vi "CompileReadHDF5PulseSeq.vi"(11 "path":path) -> (2 "parameter_config":string, 3 "pulse_seq_out":string)   [LabVIEW 2019]
uses:
  <vilib>/UPVI/lvhdf5/file.llb/LVH5F Operation.ctl
  <vilib>/UPVI/lvhdf5/group.llb/OpenCreateGroup (String).vi
  <vilib>/UPVI/lvhdf5/attribute.llb/Simple H5Aread (Variant).vi
  <vilib>/UPVI/lvhdf5/Attribute.llb/Simple H5Aread.xnode
  <vilib>/UPVI/lvhdf5/library.llb/HDF5 Ref.ctl
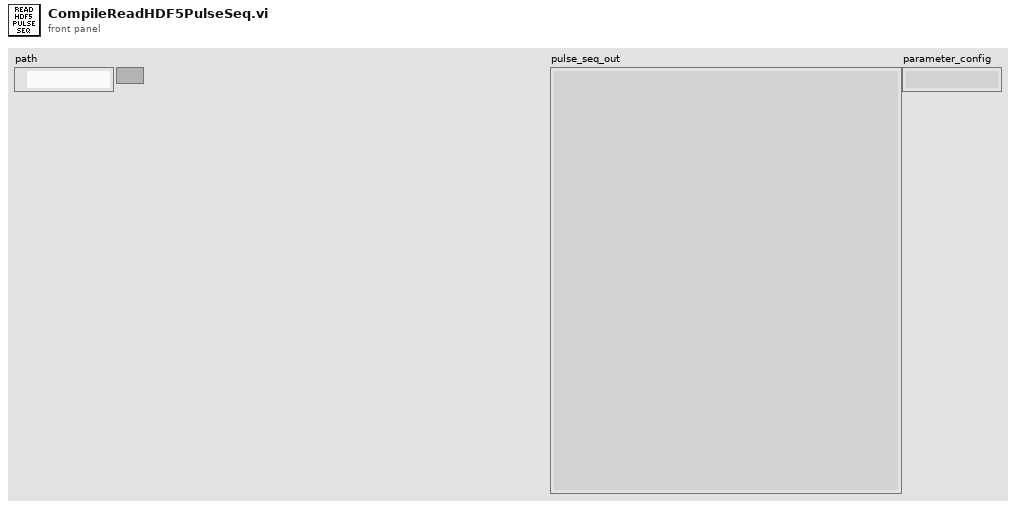
[diagram p1: front panel]
types:
  T1 = typedef "LVH5F Operation.ctl" = enum16{"open", "open or create", "create or replace", "create or replace (with confirmation)", "create", "open (read only)"}
  T2 = typedef "HDF5 Ref.ctl" = refnum<k1>
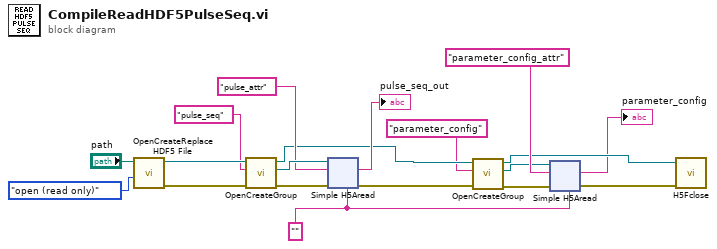
[diagram p0: block diagram]
diagram:
  w2 = ""
  n1 = call <vilib>:"OpenCreateReplace HDF5 File.vi"("function (open or create)"=LVH5F_Operation."open (read only)", "path"="path") -> ("error out"=w16:errorcluster, "HDF5 Ref out"=w17:T2)  [unwired: 6 in]
  n2 = call-poly <vilib>:"OpenCreateGroup.vi"("error in (no error)"=w16, "Group"="pulse_seq", "HDF5 Ref"=w17) -> ("error out"=w14:errorcluster, "HDF5 Group Ref"=w13:T2, "HDF5 Ref out"=w9:T2)  [unwired: 6 in]
  n3 = xnode "Simple H5Aread"("HDF5 Ref"=w13, "Name"="pulse_attr", "error in (no error)"=w14, "Type"=w2) -> ("error out"=w10:errorcluster, "Value"=→"pulse_seq_out":string)  [unwired: 1 out]
  n4 = call-poly <vilib>:"OpenCreateGroup.vi"("error in (no error)"=w10, "Group"="parameter_config", "HDF5 Ref"=w9) -> ("error out"=w7:errorcluster, "HDF5 Group Ref"=w4:T2, "HDF5 Ref out"=w3:T2)  [unwired: 6 in]
  n5 = xnode "Simple H5Aread"("HDF5 Ref"=w4, "Name"="parameter_config_attr", "error in (no error)"=w7, "Type"=w2) -> ("error out"=w6:errorcluster, "Value"=→"parameter_config":string)  [unwired: 1 out]
  n6 = call <vilib>:"H5Fclose.vi"("error in (no error)"=w6, "HDF5 Ref"=w3) -> ()  [unwired: 7 in, 1 out]
